vi "datum to filepathver2.vi"(4 "error in (no error)":errorcluster, 6 "prefix":string="C:\\Data\\ECG\\") -> (0 "error out":errorcluster, 2 "file path":path=path "C:/Data/ECG/20052801.dat")   [LabVIEW 2022 SP3]
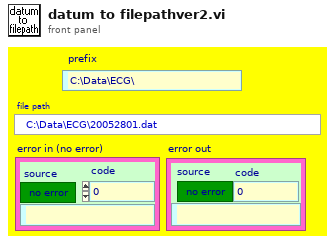
[diagram p1: front panel]
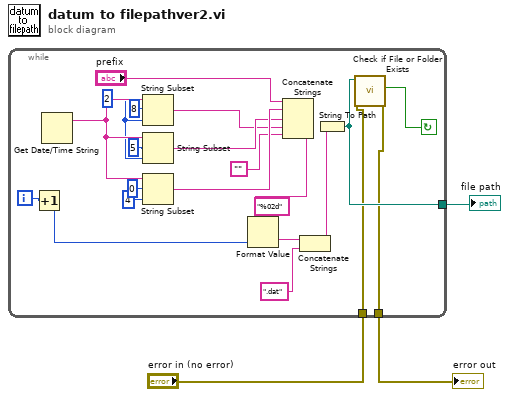
[diagram p0: block diagram]
diagram:
  n1 = while {
    tunnel: [w7] -> w3
    tunnel: "error in (no error)" -> [w6]
    tunnel: [w5] -> w1
    i -> [w16]
    stop <- w4 continue-if-true
    w24 = 2
    n2 = Increment(x=w16) -> (x+1=w11:i32)
    n3 = Get Date/Time String() -> (date string=w25:string)  [unwired: 3 in, 1 out]
    n4 = String Subset(string=w25, offset (0)=8, length (rest)=w24) -> (substring=w18:string)
    n5 = String Subset(string=w25, offset (0)=5, length (rest)=w24) -> (substring=w19:string)
    n6 = String Subset(string=w25, offset (0)=0, length (rest)=4 ("length (rest)")) -> (substring=w20:string)
    n7 = Concatenate Strings("prefix", w20, w19, w18, "") -> (w12:string)
    n8 = Format Value(string ("")=w12, format string="%02d", value (0)=w11) -> (output string=w13:string)
    n9 = Concatenate Strings(w13, ".dat") -> (w9:string)
    n10 = String To Path(string=w9) -> (path=w7:path)
    n11 = call <vilib>:"Check if File or Folder Exists.vi"("error in (no error)"=w6, "path"=w7) -> ("error out"=w5:errorcluster, "file or folder exists?"=w4:bool)  [unwired: 7 in, 1 out]
  }
  "file path" <- w3
  "error out" <- w1
